vi "ATE_BSE_MAIN.vi"(8 "Error In":errorcluster) -> (0 "Error Out":errorcluster)   [LabVIEW 2021]
uses:
  Exit Event Handler/Controls/Exit Event Handle Comamnd.ctl
  Controls/ATE_BSE_Event_type_def.ctl
  Controls/ATE_BSE_Controls_ref.ctl
  Controls/ATE_BSE_ref_type_Def.ctl
  SubVI's/IP Simulation/Controls/IP_Cellular Tech Type def.ctl
  SubVI's/IP Simulation/Controls/IP_Network_Type def.ctl
  SubVI's/IP Simulation/Controls/IP_Type-Tydedef.ctl
  Controls/ATE_BSE_Queue_Operations.ctl
  APIs/Controls/TCP_FGV.ctl
  APIs/Controls/Base_Station_Emulator.ctl
  RE HIL/RE_Main/RE TCU HIL/Modules/Manual Mode/ATE_GE_Manual Mode_VI Ref Global Variable.vi
panel:
  in  "Configurations":enum32{"Configurations", "Main"}(tab)=enum."Main"
  in  "Configure":bool
  in  "Band":enum32{"GSM", "eNodeB", "gNodeB"}(tab)
  in  "GSM-Data":enum32{"SDR", "CELL", "PHY", "GPRS"}(tab)
  in  "GSM-SDR":T1={"DL Reference Power"=-13, "Serial Name"="", "UL Reference Power"=-13, "Radio Device"="0"} {"UL Reference Power" min=-64 max=-13; "DL Reference Power" min=-64 max=-13}
  in  "GSM-CELL":T2={"SMS Enabled"="0", "Eutra Operating Bands"="850", "Power Offset Indicator"="0", "Early Classmark Sending Control"="0", "Location Area Code"=1, "CALL Enabled"="0", "Loop Back Enabled"="1", "GPRS Enabled"="0", "SI Type 2 ter Indicator"="1", "ARFCN"=0, "Frequency Format ID"=71, "Mobile Country Code"=1, "Mobile Network Code"=1, "Cell Barred Access"="0", "Downlink Frequency"=0, "Uplink Frequency"=900200000} {"Mobile Network Code" min=0 max=999; "Mobile Country Code" min=0 max=99; "Frequency Format ID" min=0 max=1024; "ARFCN" min=0 max=1023; "Location Area Code" min=0 max=65535}
  in  "GSM-PHY":T3={"RACH Maximum Retransmission"="1", "RACH Transmission Slots"="14", "RACH Call Reestablishment"="1", "RACH Access Control Class"="0", "Block for Access Grant"="2", "Multiframe for Paging"="0", "Power Control Indicator"="0", "Radio Link Timeout"="15", "Cell Reselect Hysterisis"="3", "Attach/Detach Allowed"="1", "CCCH Combinations"="1", "t3212"=0, "DTX Indicator"="1", "Power Control Level"=0, "Minimum Received Signal Level"=0, "Half Rate Support"="0", "Add Reselect"="0"} {"Minimum Received Signal Level" min=0 max=63; "Power Control Level" min=0 max=31; "t3212" min=0 max=255}
  in  "GSM-GPRS":T4={"Priority Access THR"="6", "Acess Burst Type"="0", "Nack Countdown"="8", "BCCH/PDCH Measurement"="0", "Routing Area Code(RAC)"=128, "Network Control Order"="0", "t3168"="3", "t3192"="2", "Alpha"="10"}
  in  "eNodeB-Data":enum32{"SDR", "CELL", "PHY", "RRC"}(tab)
  in  "LTE-SDR":T5={"Radio Device"="0", "DL Reference Power"=-13, "Serail Name"="", "UL Reference Power"=-13, "DL Antennas"="1", "UL Antennas"="1"} {"UL Reference Power" min=-64 max=-13; "DL Reference Power" min=-64 max=-13}
  in  "LTE-CELL":T6={"Duplex Mode"="0", "Measurement Report"="1", "Eutra Operating Bands"="3", "Carrier Bandwidth"="10", "Physical Cell ID"=0, "Network Name"="MaxEye", "DL Frequency"=1842, "UL Frequency"=1747, "Transmission Mode"="TM1", "MNC Length"="2", "IMS Enabled"="0", "Tracking Area Code"=1, "Mobile Network Code"=1, "Mobile Country Code"=1} {"Mobile Country Code" min=0 max=99; "Mobile Network Code" min=0 max=999; "Tracking Area Code" min=0 max=65535; "Physical Cell ID" min=0 max=503}
  in  "LTE-PHY":T7={"PBCH Repetition"="0", "PUCCH Delta Shift"="1", "PUCCH CQI Number of RB"="0", "PHICH Resource"="ONESIXTH", "SRS Enable"="0", "PCCH Paging Cycle"="256", "BCCH Modification Coefficient"="2", "PUSCH Alpha"="1", "PUSCH DMRS Enable"="0", "PHICH Duration"="0", "PUCCH HARQ Max Transmission"=4, "PCCH Narrowband Count"="2", "PUSCH Power Offset"=-96, "PUCCH Power Offset"=-96, "PDSCH Power Boost"="0", "PUCCH An Occassions"="0", "PUUCH CS Antenna Ports"="1", "PRACH Response Window Size"="10", "PRACH Contention Resolution Timer"="48", "PRACH Ramping Step Size"="4", "PDSCH Reference Power"=-27, "PRACH Root Sequence Index"=0, "PRACH Maximum Transmissions"="10", "PRACH Initial Received Target Power"="-108", "PRACH Configuration Index"=0} {"PRACH Configuration Index" min=0 max=63; "PRACH Root Sequence Index" min=0 max=837; "PDSCH Reference Power" min=-70 max=0; "PUCCH Power Offset" min=-127 max=-96; "PUSCH Power Offset" min=-126 max=24; "PUCCH HARQ Max Transmission" min=0 max=16}
  in  "LTE-RRC":T8={"RLC Maximum Retransmision Threshold"="4", "RLC Timer Poll Retransmit"=80, "RLC Timer Reordering"=35, "RLC Timer Status Prohibit"=0, "RLC Poll PDU"=4, "RLC Poll Byte"=25} {"RLC Poll Byte" min=0 step=25; "RLC Poll PDU" min=0 step=4; "RLC Timer Status Prohibit" min=0 max=500 step=5; "RLC Timer Reordering" min=0 max=200 step=5; "RLC Timer Poll Retransmit" min=0 max=500 step=5}
  in  "gNodeB-Data":enum32{"SDR", "CELL", "PHY", "RRC"}(tab)
  in  "NR-SDR":T9={"DL Reference Power"=-13, "Serail Name"="", "UL Reference Power"=-13, "DL Antennas"="1", "UL Antennas"="1", "Radio Device"="0"} {"UL Reference Power" min=-64 max=-13; "DL Reference Power" min=-64 max=-13}
  in  "NR-CELL":T10={"Tracking Area Code"=1, "Mobile Country Code"=1, "Mobile Network Code"=1, "Operating Bands"="77", "Physical Cell ID"=0, "DL Offset to Carrier"=0, "Subcarrier Spacing"="1", "UL Offset to Carrier 2"=0, "Carrier Bandwidth"="10", "Transmission Mode"="TM1", "CSI-RS"="1", "SRS"="1", "Measurement Report"="1"} {"Physical Cell ID" min=0 max=503; "Mobile Network Code" min=0 max=999; "Mobile Country Code" min=0 max=99; "Tracking Area Code" min=0 max=65535}
  in  "NR-PHY":T11={"PDSCH Reference Power"=-27, "SSB RSRP Threshold"=-109, "PRACH Contention Resolution Timer"=7, "Preamble Per SSB"=14, "Preamble Per SSB Format"=4, "UE Power Level Grant"=-90, "RA Response Window"="10", "Power Ramp Step Size"="2", "Preamble Root Sequence Index"="139", "Preamble Transmission Count"="10", "Preamble Received Power"=-96, "Zero Correlation Zone Configuration"=13, "Msg Frequency Division Multiplexing"="one", "PRACH Configuration Index"=98, "Preamble Timing Offset"=1, "Preamble Format"=0, "Resource Restriction Type"="0"} {"Preamble Format" min=0 max=3; "Preamble Timing Offset" min=-1 max=6; "PRACH Configuration Index" min=0 max=255; "Zero Correlation Zone Configuration" min=1 max=15; "Preamble Received Power" min=-202 max=-60; "UE Power Level Grant" min=-202 max=24; "Preamble Per SSB Format" min=0 max=7; "Preamble Per SSB" min=1 max=16; "PRACH Contention Resolution Timer" min=0 max=7; "SSB RSRP Threshold" min=-140 max=-90; "PDSCH Reference Power" min=-70 max=0}
  in  "NR-RRC":T12={"Ciphering Algorithms for SRB"="0", "Integrity Algorithms for SRB"="0", "Ciphering Algorithms for DRB"="1", "Integrity Algorithms for DRB"="1"}
  in  "Cancel Configurations":bool
  in  "Sim Configurations":bool
  in  "SelectNetwork2":cluster{"Nw1-check":bool, "NW-Combo":string}={"Nw1-check"=FALSE, "NW-Combo"="GSM"}
  in  "SelectNetwork1":cluster{"Nw1-check":bool, "NW-Combo":string}={"Nw1-check"=FALSE, "NW-Combo"="GSM"}
  in  "SelectNetwork3":cluster{"Nw1-check":bool, "NW-Combo":string}={"Nw1-check"=FALSE, "NW-Combo"="GSM"}
  in  "WWW":bool
  in  "IMS":bool
  in  "ECall":bool
  in  "UE4":bool
  in  "UE3":bool
  in  "UE2":bool
  in  "UE1":bool
  out "Trace_Table2":i32(listbox)
  out "Trace_Table1":i32(listbox)
  out "Status":string
  in  "IP simulation":bool
  in  "Start":bool
  in  "Reset":bool
  in  "Download":bool
  in  "Upload":bool
  out "UE - 4":T13
  out "UE - 3":T14
  out "UE - 2":T15
  out "UE - 1":T16
  out "Network-1":T17
  out "Network-2":T18
  out "Network-3":T19
  out "Time Stamp":timestamp format="%<%H:%M:%S>T"
  # "Cellular Network Emulator"
  # "BASE STATION :"
  # "CONFIGURATIONS"
  # "Power Level"
  # "Frequency"
  # "Throughput"
  # "Downlink"
  # "Uplink"
  # "NETWORK - 1"
  # "Power Level"
  # "Frequency"
  # "Throughput"
  # "Downlink"
  # "Uplink"
  # "NETWORK - 2"
  # "Power Level"
  # "Frequency"
  # "Throughput"
  # "Downlink"
  # "Uplink"
  # "NETWORK - 3"
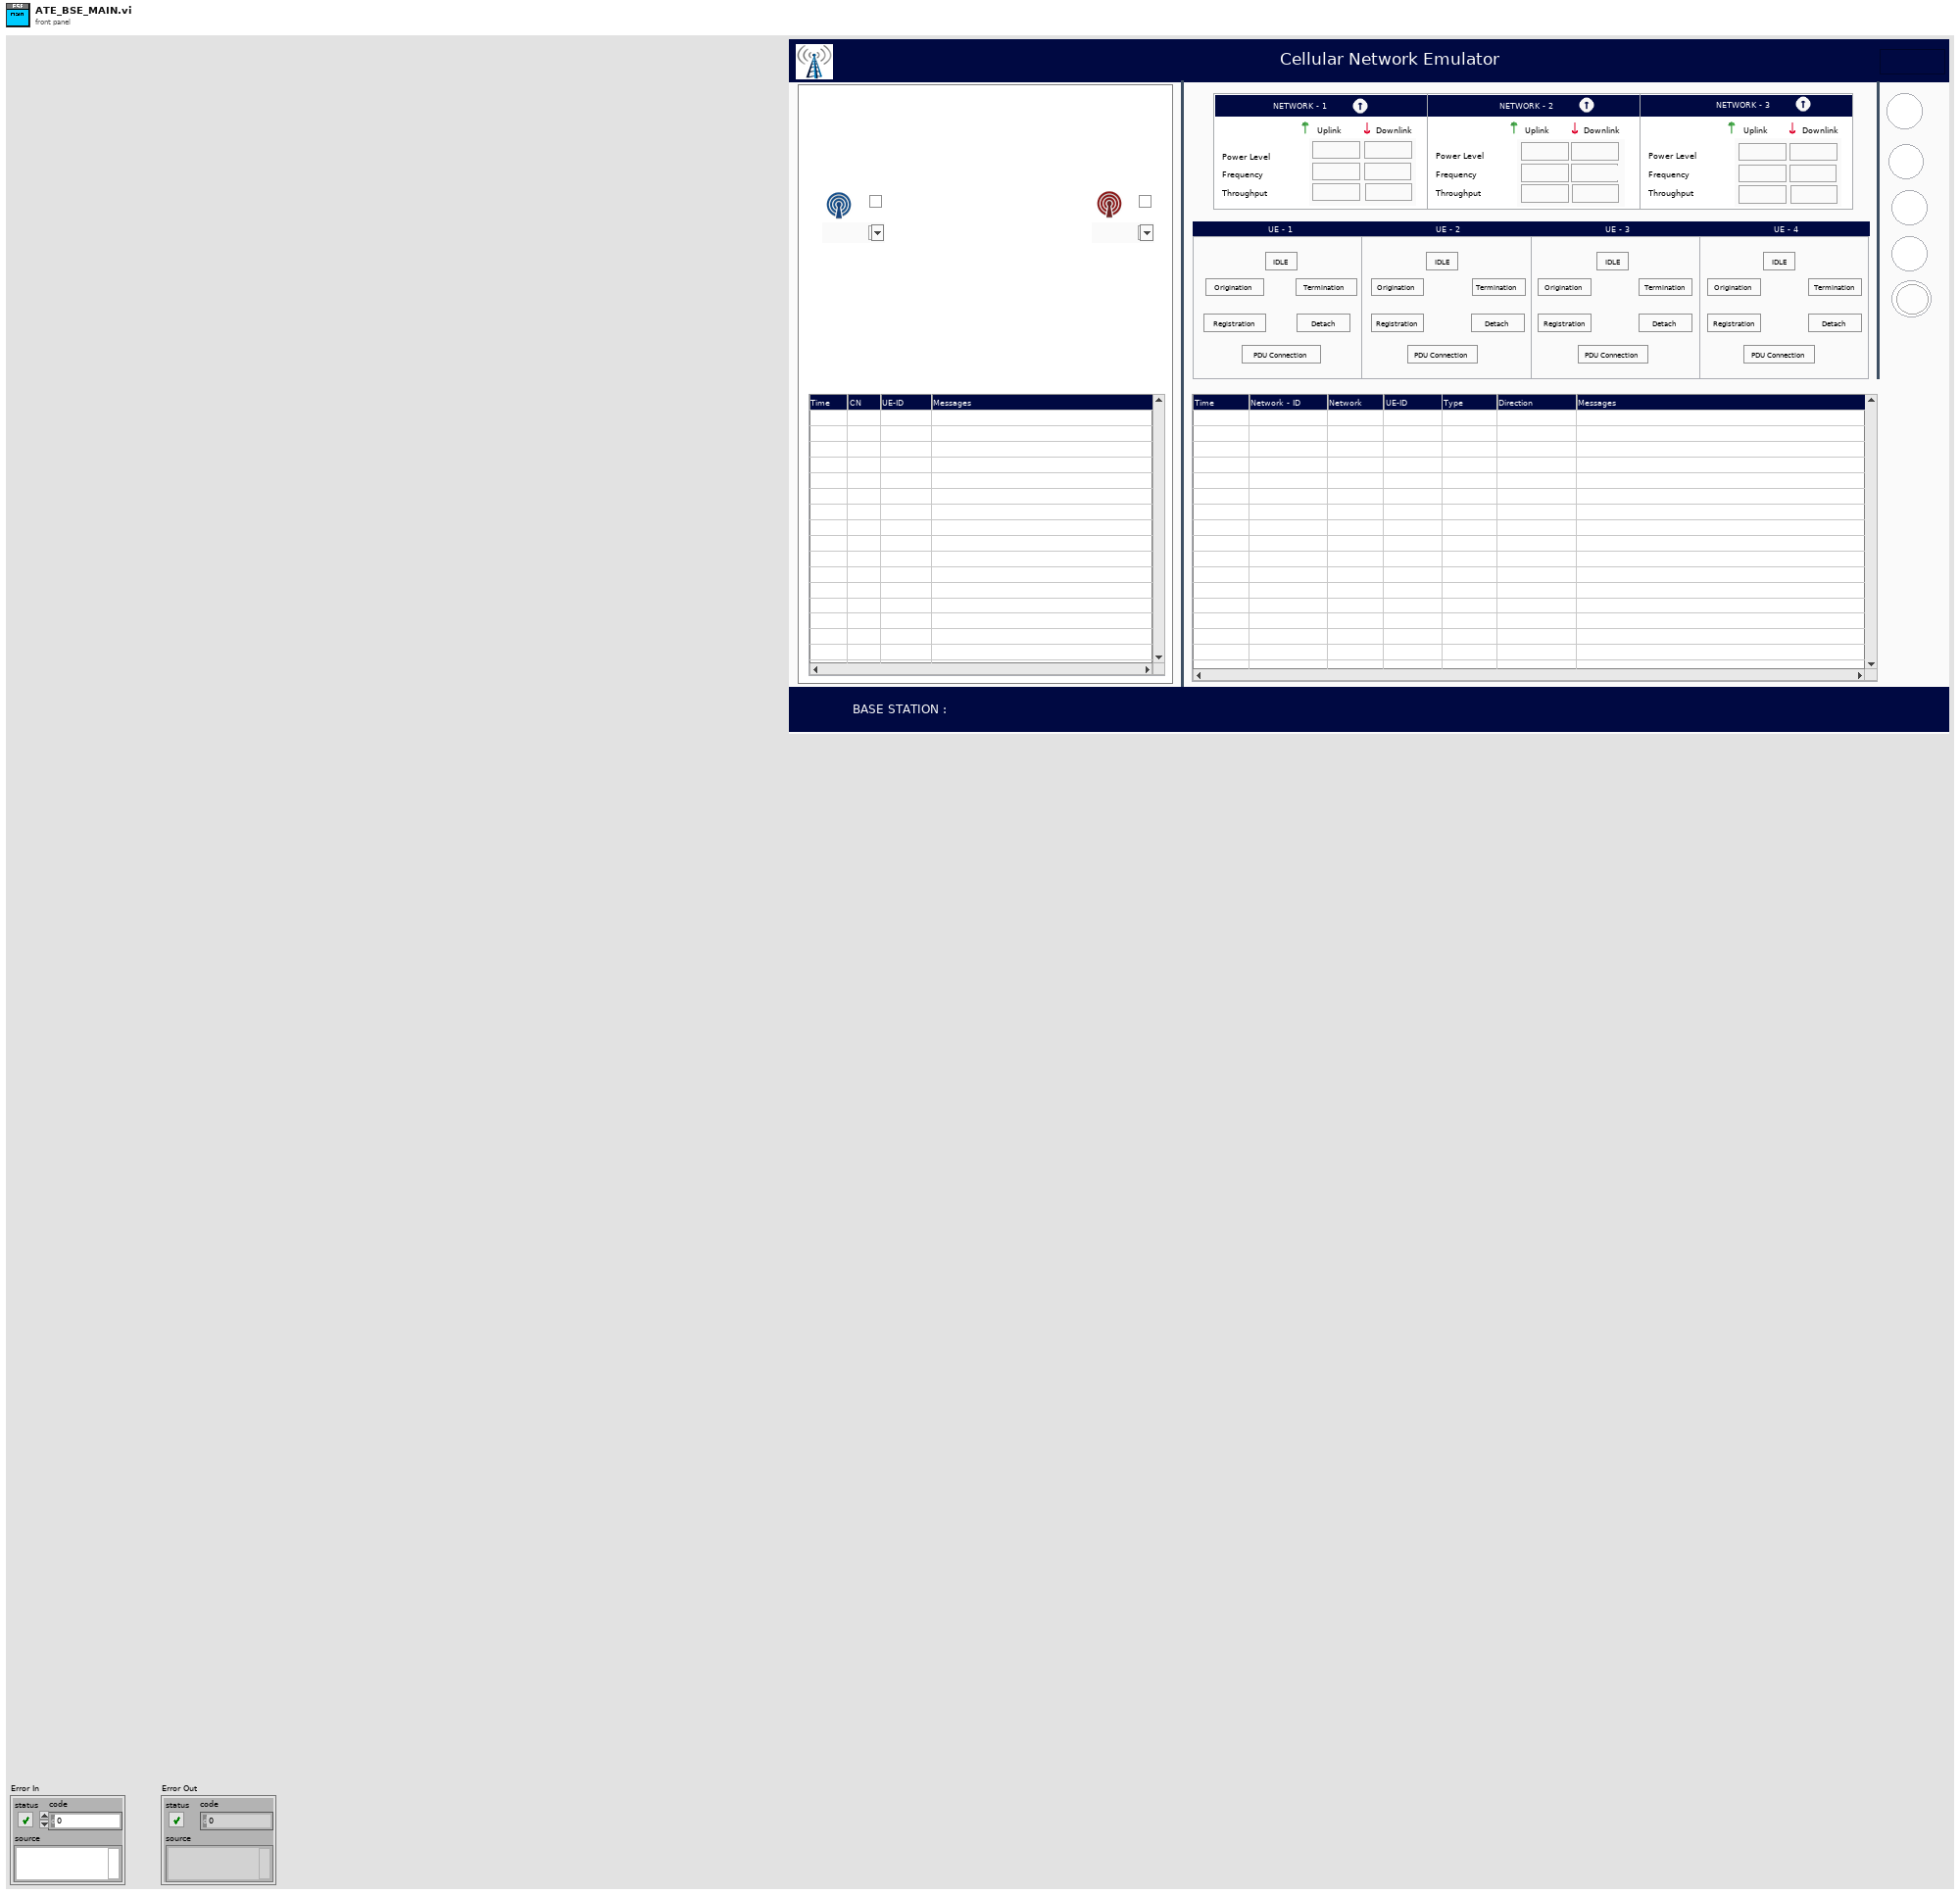
[diagram p1: front panel]
types:
  T1 = cluster{"DL Reference Power":i32, "Serial Name":string, "UL Reference Power":i32, "Radio Device":string}
  T2 = cluster{"SMS Enabled":string, "Eutra Operating Bands":string, "Power Offset Indicator":string, "Early Classmark Sending Control":string, "Location Area Code":i32, "CALL Enabled":string, "Loop Back Enabled":string, "GPRS Enabled":string, "SI Type 2 ter Indicator":string, "ARFCN":i64, "Frequency Format ID":i64, "Mobile Country Code":i64, "Mobile Network Code":i64, "Cell Barred Access":string, "Downlink Frequency":i32, "Uplink Frequency":i32}
  T3 = cluster{"RACH Maximum Retransmission":string, "RACH Transmission Slots":string, "RACH Call Reestablishment":string, "RACH Access Control Class":string, "Block for Access Grant":string, "Multiframe for Paging":string, "Power Control Indicator":string, "Radio Link Timeout":string, "Cell Reselect Hysterisis":string, "Attach/Detach Allowed":string, "CCCH Combinations":string, "t3212":i64, "DTX Indicator":string, "Power Control Level":i64, "Minimum Received Signal Level":i64, "Half Rate Support":string, "Add Reselect":string}
  T4 = cluster{"Priority Access THR":string, "Acess Burst Type":string, "Nack Countdown":string, "BCCH/PDCH Measurement":string, "Routing Area Code(RAC)":i32, "Network Control Order":string, "t3168":string, "t3192":string, "Alpha":string}
  T5 = cluster{"Radio Device":string, "DL Reference Power":i32, "Serail Name":string, "UL Reference Power":i32, "DL Antennas":string, "UL Antennas":string}
  T6 = cluster{"Duplex Mode":string, "Measurement Report":string, "Eutra Operating Bands":string, "Carrier Bandwidth":string, "Physical Cell ID":i64, "Network Name":string, "DL Frequency":i32, "UL Frequency":i32, "Transmission Mode":string, "MNC Length":string, "IMS Enabled":string, "Tracking Area Code":i32, "Mobile Network Code":i32, "Mobile Country Code":i32}
  T7 = cluster{"PBCH Repetition":string, "PUCCH Delta Shift":string, "PUCCH CQI Number of RB":string, "PHICH Resource":string, "SRS Enable":string, "PCCH Paging Cycle":string, "BCCH Modification Coefficient":string, "PUSCH Alpha":string, "PUSCH DMRS Enable":string, "PHICH Duration":string, "PUCCH HARQ Max Transmission":i64, "PCCH Narrowband Count":string, "PUSCH Power Offset":i64, "PUCCH Power Offset":i64, "PDSCH Power Boost":string, "PUCCH An Occassions":string, "PUUCH CS Antenna Ports":string, "PRACH Response Window Size":string, "PRACH Contention Resolution Timer":string, "PRACH Ramping Step Size":string, "PDSCH Reference Power":i64, "PRACH Root Sequence Index":i64, "PRACH Maximum Transmissions":string, "PRACH Initial Received Target Power":string, "PRACH Configuration Index":i64}
  T8 = cluster{"RLC Maximum Retransmision Threshold":string, "RLC Timer Poll Retransmit":i32, "RLC Timer Reordering":i32, "RLC Timer Status Prohibit":i32, "RLC Poll PDU":i32, "RLC Poll Byte":i32}
  T9 = cluster{"DL Reference Power":i32, "Serail Name":string, "UL Reference Power":i32, "DL Antennas":string, "UL Antennas":string, "Radio Device":string}
  T10 = cluster{"Tracking Area Code":i64, "Mobile Country Code":i64, "Mobile Network Code":i64, "Operating Bands":string, "Physical Cell ID":i64, "DL Offset to Carrier":i32, "Subcarrier Spacing":string, "UL Offset to Carrier 2":i32, "Carrier Bandwidth":string, "Transmission Mode":string, "CSI-RS":string, "SRS":string, "Measurement Report":string}
  T11 = cluster{"PDSCH Reference Power":i64, "SSB RSRP Threshold":i64, "PRACH Contention Resolution Timer":i64, "Preamble Per SSB":i64, "Preamble Per SSB Format":i64, "UE Power Level Grant":i64, "RA Response Window":string, "Power Ramp Step Size":string, "Preamble Root Sequence Index":string, "Preamble Transmission Count":string, "Preamble Received Power":i64, "Zero Correlation Zone Configuration":i64, "Msg Frequency Division Multiplexing":string, "PRACH Configuration Index":i64, "Preamble Timing Offset":i64, "Preamble Format":i64, "Resource Restriction Type":string}
  T12 = cluster{"Ciphering Algorithms for SRB":string, "Integrity Algorithms for SRB":string, "Ciphering Algorithms for DRB":string, "Integrity Algorithms for DRB":string}
  T13 = cluster{"UE4-Idle":bool, "UE4-Origination":bool, "UE4-Registration":bool, "UE4-Pdu Connection":bool, "UE4-Termination":bool, "UE4-Detach":bool}
  T14 = cluster{"UE3-Idle":bool, "UE3-Origination":bool, "UE3-Registration":bool, "UE3-Pdu Connection":bool, "UE3-Termination":bool, "UE3-Detach":bool}
  T15 = cluster{"UE2-Idle":bool, "UE2-Origination":bool, "UE2-Registration":bool, "UE2-Pdu Connection":bool, "UE2-Termination":bool, "UE2-Detach":bool}
  T16 = cluster{"UE1-Idle":bool, "UE1-Origination":bool, "UE1-Registration":bool, "UE1-Pdu Connection":bool, "UE1-Termination":bool, "UE1-Detach":bool}
  T17 = cluster{"NW1-Thr-Down":dbl, "NW1-Thr-Up":dbl, "NW1-Fre-Down":dbl, "NW1-Fre-Up":dbl, "NW1-PwL-Down":dbl, "NW1-PwL-Up":dbl}
  T18 = cluster{"NW2-Thr-Down":dbl, "NW2-Thr-Up":dbl, "NW2-Fre-Down":dbl, "NW2-Fre-Up":dbl, "NW2-PwL-Down":dbl, "NW2-PwL-Up":dbl}
  T19 = cluster{"NW3-Thr-Down":dbl, "NW3-Thr-Up":dbl, "NW3-Fre-Down":dbl, "NW3-Fre-Up":dbl, "NW3-PwL-Down":dbl, "NW3-PwL-Up":dbl}
  T20 = typedef "ATE_BSE_Queue_Operations.ctl" = enum16{"Init", "Get Queue", "Flush", "Close"}
  T21 = typedef "ATE_BSE_Controls_ref.ctl" = cluster{"Ref_Cluster":T22, "Time Stamp":timestamp, "Network-3":cluster{"NW3-Thr-Down":dbl, "NW3-Thr-Up":dbl, "NW3-Fre-Down":dbl, "NW3-Fre-Up":dbl, "NW3-PwL-Down":dbl, "NW3-PwL-Up":dbl}, "Network-2":cluster{"NW2-Thr-Down":dbl, "NW2-Thr-Up":dbl, "NW2-Fre-Down":dbl, "NW2-Fre-Up":dbl, "NW2-PwL-Down":dbl, "NW2-PwL-Up":dbl}, "Network-1":cluster{"NW1-Thr-Down":dbl, "NW1-Thr-Up":dbl, "NW1-Fre-Down":dbl, "NW1-Fre-Up":dbl, "NW1-PwL-Down":dbl, "NW1-PwL-Up":dbl}, "UE - 4":cluster{"UE4-Idle":bool, "UE4-Origination":bool, "UE4-Registration":bool, "UE4-Pdu Connection":bool, "UE4-Termination":bool, "UE4-Detach":bool}, "UE - 2":cluster{"UE2-Idle":bool, "UE2-Origination":bool, "UE2-Registration":bool, "UE2-Pdu Connection":bool, "UE2-Termination":bool, "UE2-Detach":bool}, "UE - 1":cluster{"UE1-Idle":bool, "UE1-Origination":bool, "UE1-Registration":bool, "UE1-Pdu Connection":bool, "UE1-Termination":bool, "UE1-Detach":bool}, "UE - 3":cluster{"UE3-Idle":bool, "UE3-Origination":bool, "UE3-Registration":bool, "UE3-Pdu Connection":bool, "UE3-Termination":bool, "UE3-Detach":bool}, "IP simulation":bool, "Stop":bool, "Reset":bool, "Download":bool, "Upload":bool, "UE4":bool, "UE3":bool, "UE2":bool, "UE1":bool, "Trace_Table1":i32, "Status":string, "Trace_Table2":i32, "SelectNetwork1":cluster{"Nw1-check":bool, "NW-Combo":string}, "SelectNetwork2":cluster{"Nw1-check":bool, "NW-Combo":string}, "SelectNetwork3":cluster{"Nw1-check":bool, "NW-Combo":string}, "IMS":bool, "WWW":bool, "Sim Configuration":bool, "Ecall":bool, "Configurations":enum32{"Configurations", "Main"}, "Band":enum32{"GSM", "gNodeB", "eNodeB"}, "GSM-Data":enum32{"SDR", "CELL", "PHY", "GPRS"}, "eNodeB-Data":enum32{"SDR", "CELL", "PHY", "RRC"}, "gNodeB-Data":enum32{"SDR", "CELL", "PHY", "RRC"}, "Cancel Configurations":bool, "GSM-SDR":cluster{"DL Reference Power":i32, "Serail Name":string, "UL Reference Power":i32, "Radio Device":string}, "GSM-PHY":cluster{"RACH Maximum Retransmission":string, "RACH Transmission Slots":string, "RACH Call Reestablishment":string, "RACH Access Control Class":string, "Block for Access Grant":string, "Multiframe for Paging":string, "Power Control Indicator":string, "Radio Link Timeout":string, "Cell Reselect Hysterisis":string, "Attach/Detach Allowed":string, "CCCH Combinations":string, "t3212":i64, "DTX Indicator":string, "Power Control Level":i64, "Minimum Received Signal Level":i64, "Half Rate Support":string, "Add Reselect":string}, "GSM-CELL":cluster{"SMS Enabled":string, "Eutra Operating Bands":string, "Power Offset Indicator":string, "Early Classmark Sending Control":string, "Location Area Code":i32, "CALL Enabled":string, "Loop Back Enabled":string, "GPRS Enabled":string, "SI Type 2 ter Indicator":string, "ARFCN":i64, "Frequency Format ID":i64, "Mobile Country Code":i64, "Mobile Network Code":i64, "Cell Barred Access":string, "Downlink Frequency":i32, "Uplink Frequency":i32}, "GSM-GPRS":cluster{"Priority Access THR":string, "Acess Burst Type":string, "Nack Countdown":string, "BCCH/PDCH Measurement":string, "Routing Area Code(RAC)":i32, "Network Control Order":string, "t3168":string, "t3192":string, "Alpha":string}, "LTE-SDR":cluster{"Radio Device":string, "DL Reference Power":i32, "Serail Name":string, "UL Reference Power":i32, "DL Antennas":string, "UL Antennas":string}, "LTE-PHY":cluster{"PBCH Repetition":string, "PUCCH Delta Shift":string, "PUCCH CQI Number of RB":string, "PHICH Resource":string, "SRS Enable":string, "PCCH Paging Cycle":string, "BCCH Modification Coefficient":string, "PUSCH Alpha":string, "PUSCH DMRS Enable":string, "PHICH Duration":string, "PUCCH HARQ Max Transmission":i64, "PCCH Narrowband Count":string, "PUSCH Power Offset":i64, "PUCCH Power Offset":i64, "PDSCH Power Boost":string, "PUCCH An Occassions":string, "PUUCH CS Antenna Ports":string, "PRACH Response Window Size":string, "PRACH Contention Resolution Timer":string, "PRACH Ramping Step Size":string, "PDSCH Reference Power":i64, "PRACH Root Sequence Index":i64, "PRACH Maximum Transmissions":string, "PRACH Initial Received Target Power":string, "PRACH Configuration Index":i64}, "LTE-CELL":cluster{"Duplex Mode":string, "Measurement Report":string, "Eutra Operating Bands":string, "Carrier Bandwidth":string, "Physical Cell ID":i64, "Network Name":string, "DL Frequency":i32, "UL Frequency":i32, "Transmission Mode":string, "MNC Length":string, "IMS Enabled":string, "Tracking Area Code":i32, "Mobile Network Code":i32, "Mobile Country Code":i32}, "LTE-RRC":cluster{"RLC Maximum Retransmision Threshold":string, "RLC Timer Poll Retransmit":i32, "RLC Timer Reordering":i32, "RLC Timer Status Prohibit":i32, "RLC Poll PDU":i32, "RLC Poll Byte":i32}, "NR-SDR":cluster{"DL Reference Power":i32, "Serail Name":string, "UL Reference Power":i32, "DL Antennas":string, "UL Antennas":string, "Radio Device":string}, "NR-PHY":cluster{"PDSCH Reference Power":i64, "SSB RSRP Threshold":i64, "PRACH Contention Resolution Timer":i64, "Preamble Per SSB":i64, "Preamble Per SSB Format":i64, "UE Power Level Grant":i64, "RA Response Window":string, "Power Ramp Step Size":string, "Preamble Root Sequence Index":string, "Preamble Transmission Count":string, "Preamble Received Power":i64, "Zero Correlation Zone Configuration":i64, "Msg Frequency Division Multiplexing":string, "PRACH Configuration Index":i64, "Preamble Timing Offset":i64, "Preamble Format":i64, "Resource Restriction Type":string}, "NR-CELL":cluster{"Tracking Area Code":i64, "Mobile Country Code":i64, "Mobile Network Code":i64, "Operating Bands":string, "Physical Cell ID":i64, "DL Offset to Carrier":i32, "Subcarrier Spacing":string, "UL Offset to Carrier 2":i32, "Carrier Bandwidth":string, "Transmission Mode":string, "CSI-RS":string, "SRS":string, "Measurement Report":string}, "NR-RRC":cluster{"Ciphering Algorithms for SRB":string, "Integrity Algorithms for SRB":string, "Ciphering Algorithms for DRB":string, "Integrity Algorithms for DRB":string}, "IP_UI":cluster{"Add":bool, "Close":bool, "IP_UI":cluster{"Cellular Tect":T23, "IP_NETWORK":T24, "IP_TYPE":T25, "IP_Client Address":string, "IP_ThgroughPut(Mbps)":i32, "Duration":i32, "Run":bool}[]}, "IMS_DATA":string[][], "ECall DATA":string[][]}
  T22 = typedef "ATE_BSE_ref_type_Def.ctl" = cluster{"UE1":refnum<vi>, "UE2":refnum<vi>, "UE3":refnum<vi>, "SelectNetwork1":refnum<vi>, "SelectNetwork3":refnum<vi>, "SelectNetwork2":refnum<vi>, "Trace_Table1":refnum<vi>, "UE - 1":refnum<vi>, "UE - 2":refnum<vi>, "UE - 3":refnum<vi>, "UE - 4":refnum<vi>, "Network-3":refnum<vi>, "Status":refnum<vi>, "Trace_Table2":refnum<vi>, "UE4":refnum<vi>, "Stop":refnum<vi>, "Reset":refnum<vi>, "IP simulation":refnum<vi>, "Upload":refnum<vi>, "Download":refnum<vi>, "Network-1":refnum<vi>, "Time Stamp":refnum<vi>, "Network-2":refnum<vi>, "IMS":refnum<vi>, "GSM-Data":refnum<vi>, "Configurations":refnum<vi>, "Band":refnum<vi>, "Sim Configurations":refnum<vi>, "ECall":refnum<vi>, "WWW":refnum<vi>, "Cancel Configurations":refnum<vi>, "GSM-PHY":refnum<vi>, "GSM-CELL":refnum<vi>, "GSM-GPRS":refnum<vi>, "LTE-CELL":refnum<vi>, "LTE-PHY":refnum<vi>, "LTE-RRC":refnum<vi>, "LTE-SDR":refnum<vi>, "NR-RRC":refnum<vi>, "NR-SDR":refnum<vi>, "NR-PHY":refnum<vi>, "NR-CELL":refnum<vi>, "GSM-SDR":refnum<vi>, "gNodeB-Data":refnum<vi>, "eNodeB-Data":refnum<vi>}
  T23 = typedef "IP_Cellular Tech Type def.ctl" = string
  T24 = typedef "IP_Network_Type def.ctl" = string
  T25 = typedef "IP_Type-Tydedef.ctl" = string
  T26 = typedef "ATE_BSE_Event_type_def.ctl" = enum16{"Initialize", "Configure", "Ip Simulation", "IMS", "ECall", "Start Base Station", "Exit", "Error"}
  T27 = typedef "Exit Event Handle Comamnd.ctl" = enum16{"Init", "Close", "Generate Event"}
  T28 = cluster{"Cellular Tect":T23, "IP_NETWORK":T24, "IP_TYPE":T25, "IP_Client Address":string, "IP_ThgroughPut(Mbps)":i32, "Duration":i32, "Run":bool}[]
  T29 = typedef "TCP_FGV.ctl" = enum16{"Open", "Read", "Write", "Close"}
  T30 = typedef "Base_Station_Emulator.ctl" = string
  T31 = cluster{"Add":bool, "Close":bool, "IP_UI":cluster{"Cellular Tect":T23, "IP_NETWORK":T24, "IP_TYPE":T25, "IP_Client Address":string, "IP_ThgroughPut(Mbps)":i32, "Duration":i32, "Run":bool}[]}
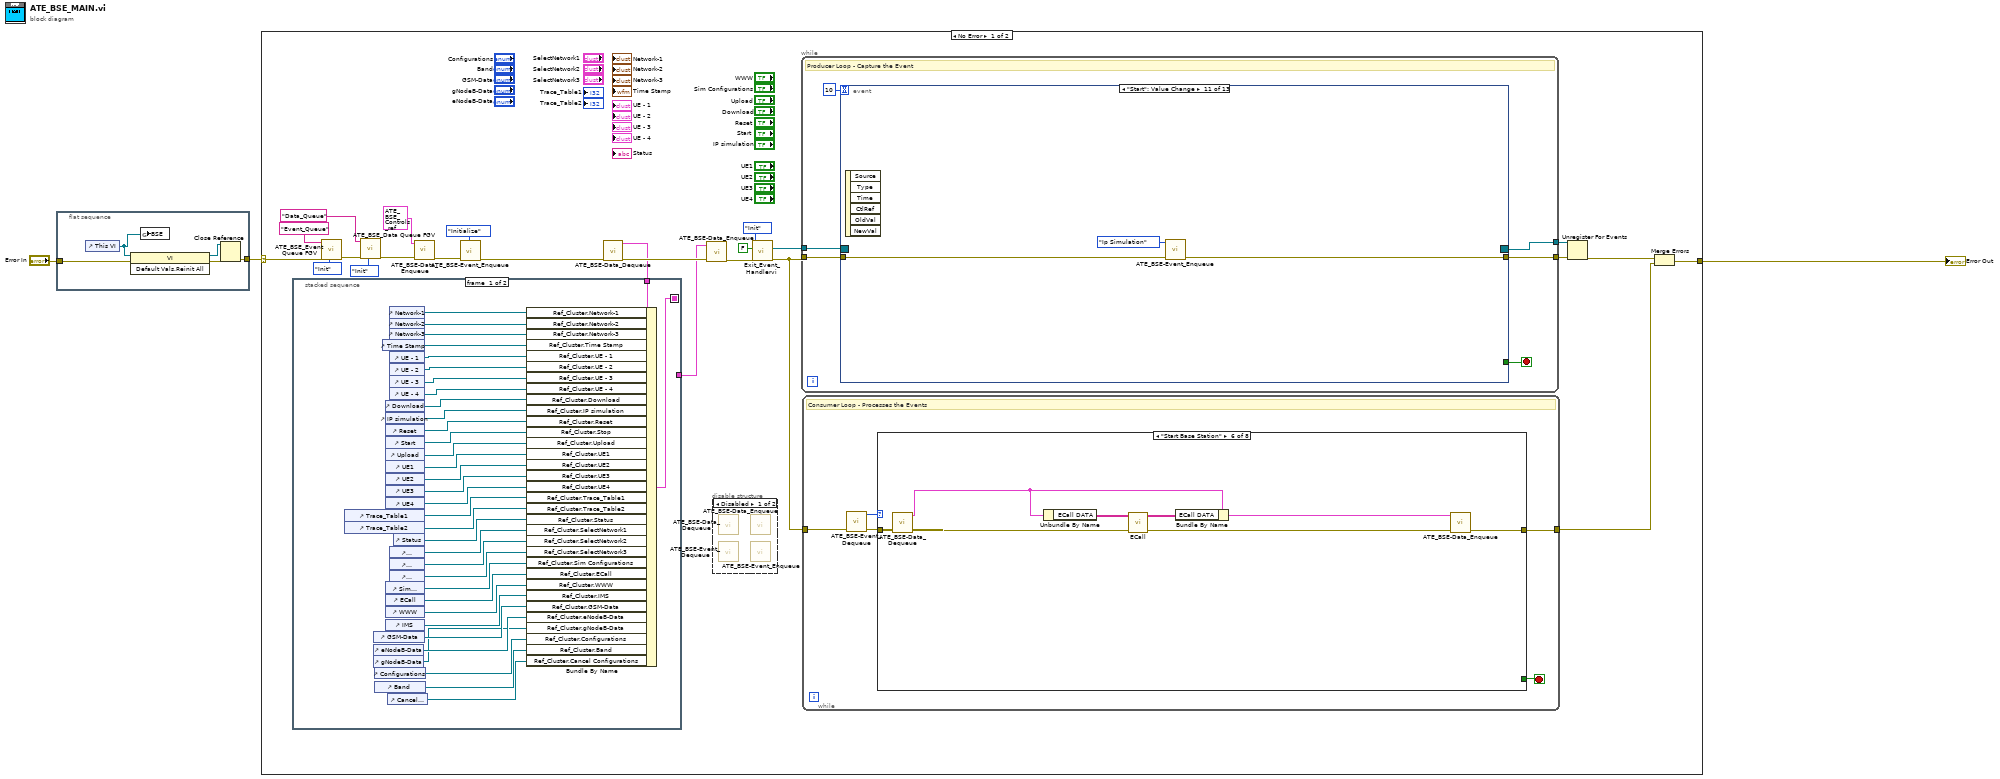
[diagram p0: block diagram]
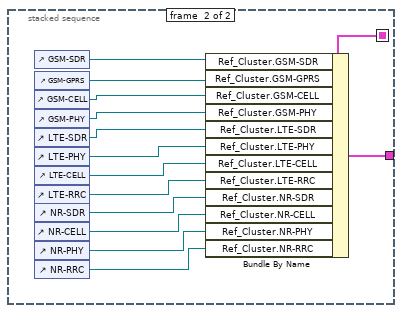
[diagram p2: hidden frame]
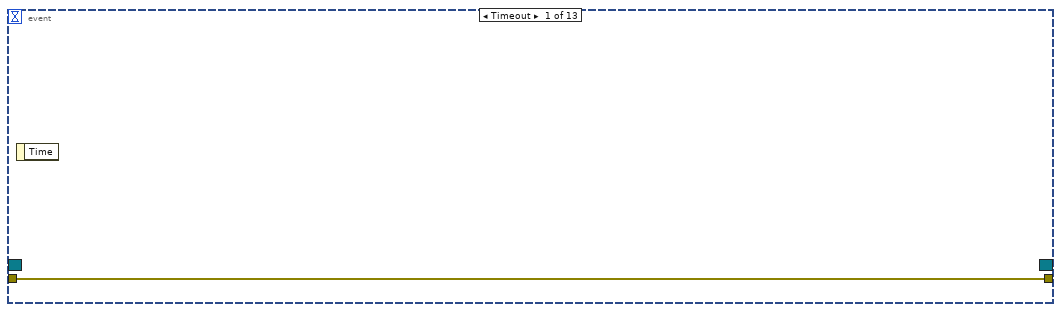
[diagram p4: hidden frame]
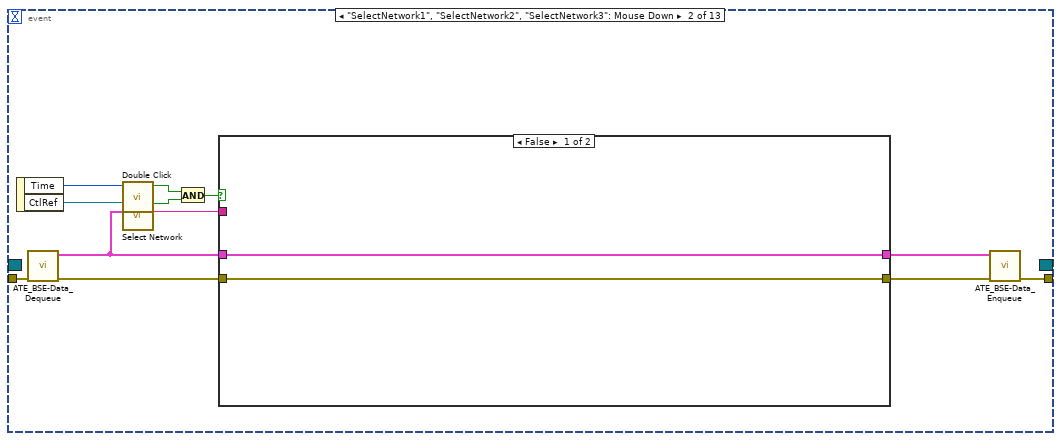
[diagram p5: hidden frame]
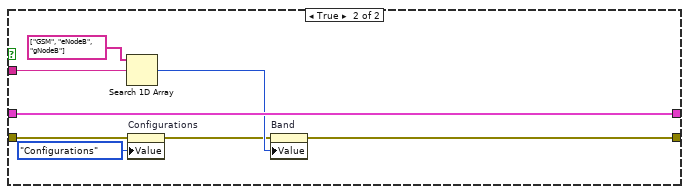
[diagram p6: hidden frame]
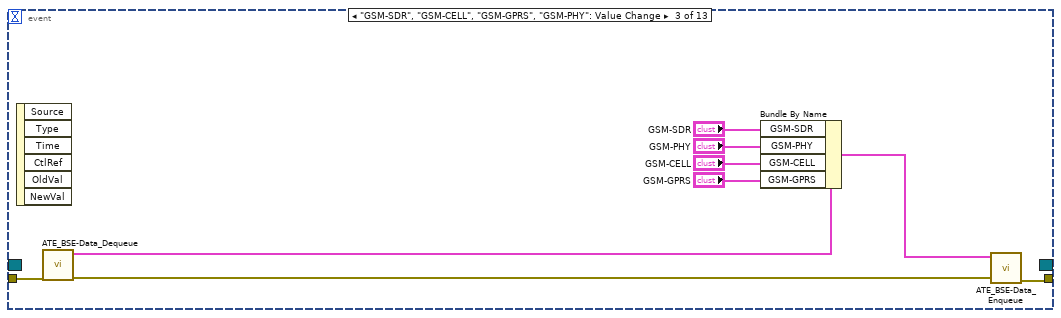
[diagram p7: hidden frame]
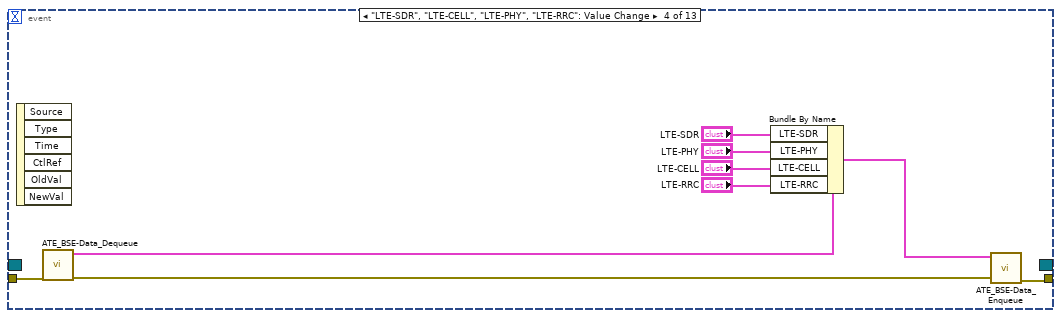
[diagram p8: hidden frame]
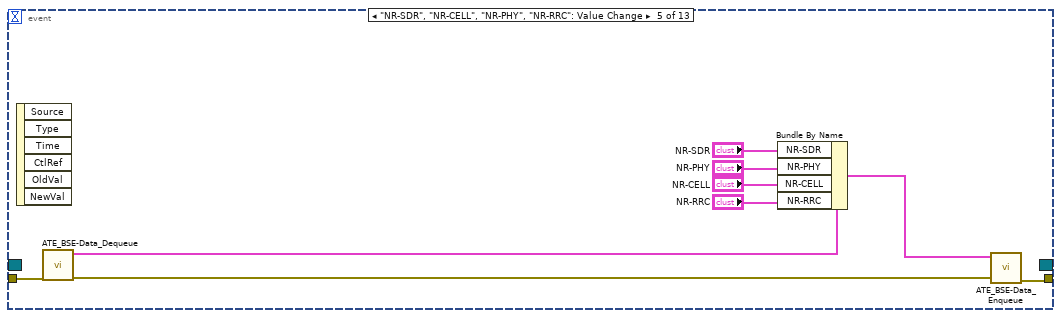
[diagram p9: hidden frame]
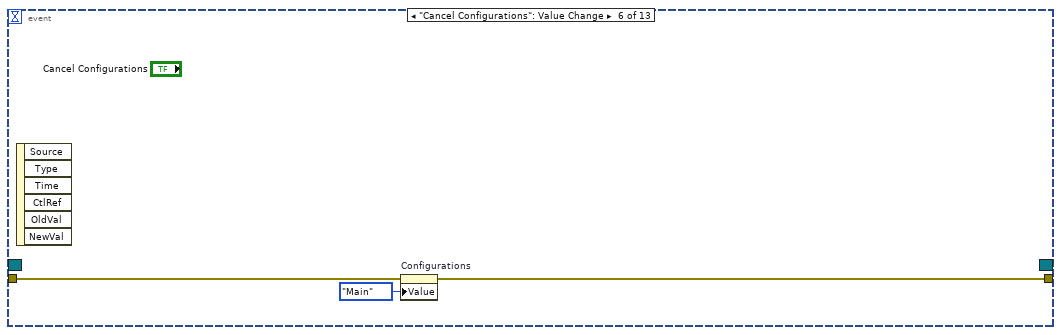
[diagram p10: hidden frame]
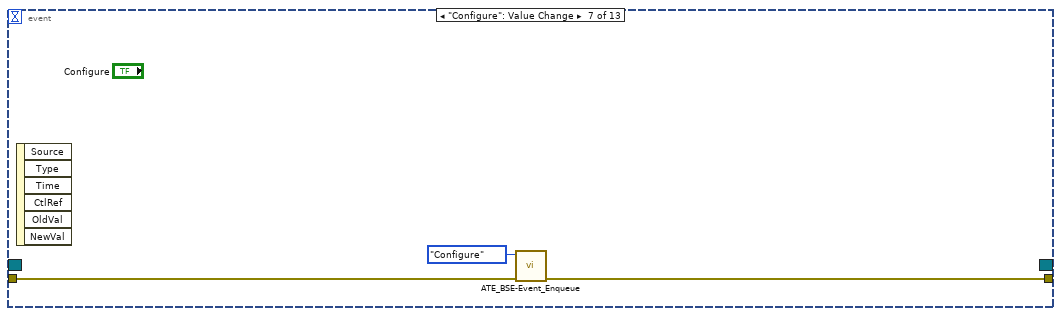
[diagram p11: hidden frame]
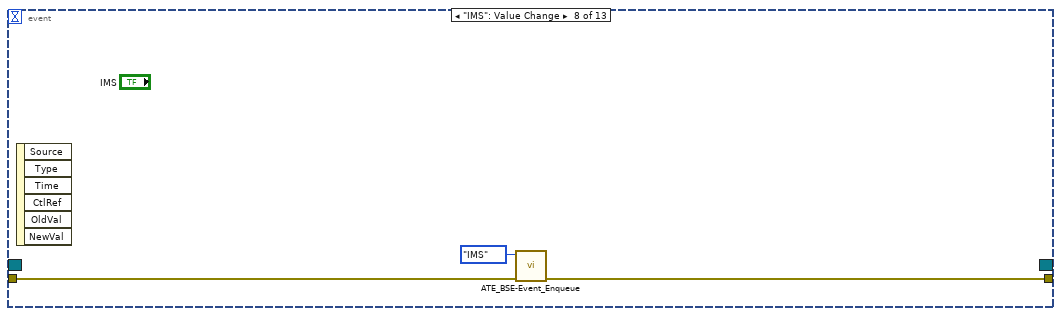
[diagram p12: hidden frame]
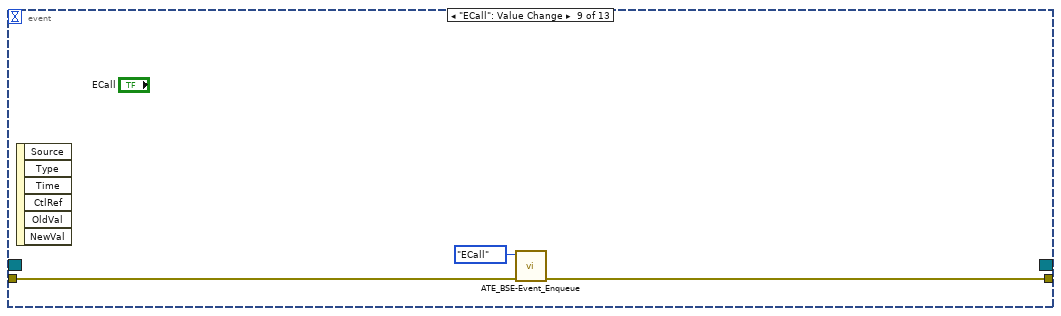
[diagram p13: hidden frame]
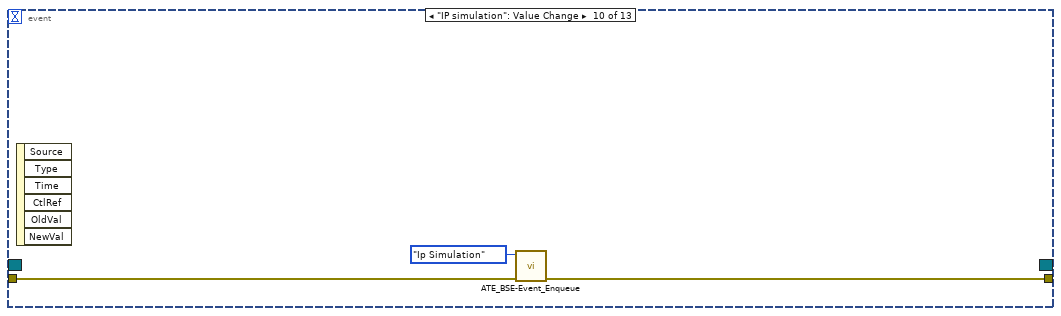
[diagram p14: hidden frame]
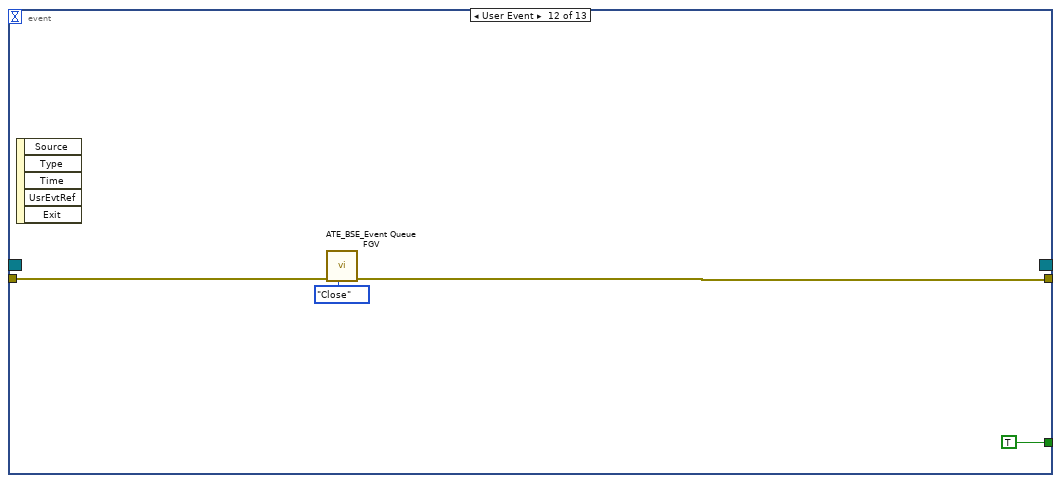
[diagram p15: hidden frame]
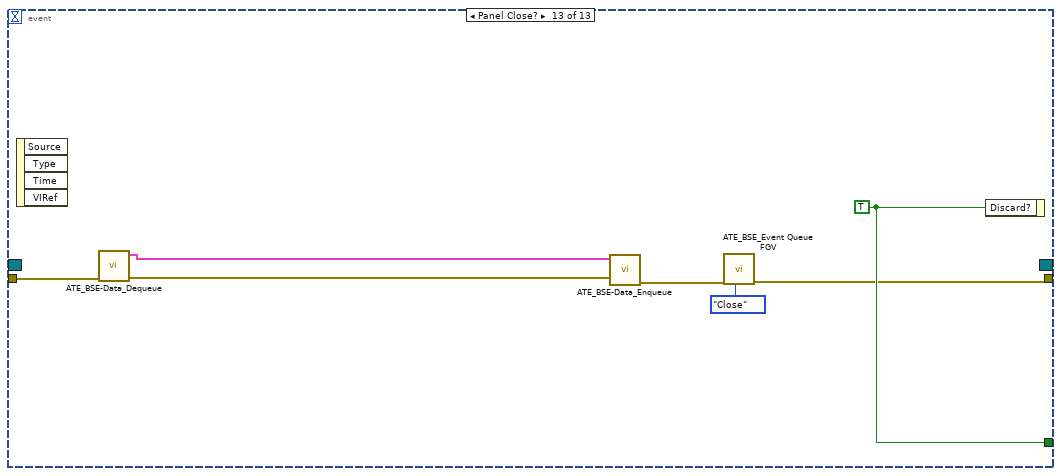
[diagram p16: hidden frame]
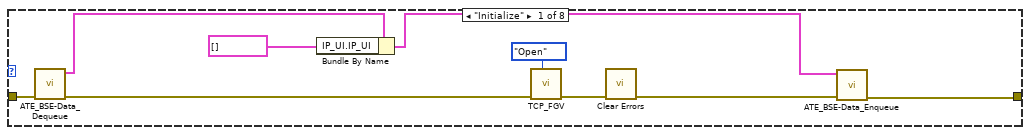
[diagram p17: hidden frame]
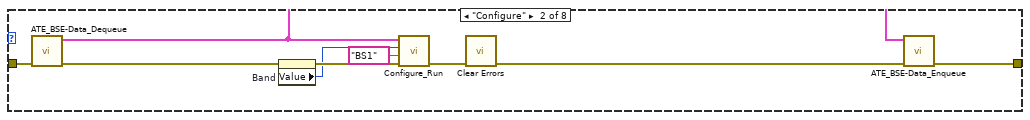
[diagram p18: hidden frame]
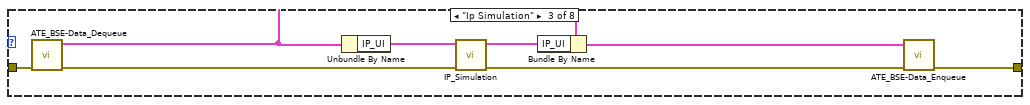
[diagram p19: hidden frame]
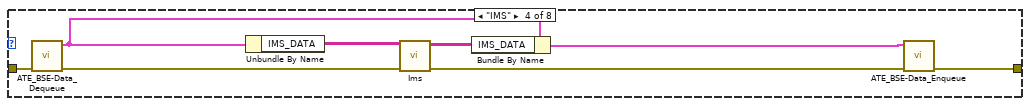
[diagram p20: hidden frame]
diagram:
  n1 = flat-sequence {
    tunnel: "Error In" -> [w6]
    tunnel: [w5] -> w1
    frame #0 {
      n2 = control-ref of="This VI"() -> (w4:refnum<vi>)
      n3 = invoke class="VI" method="Default Vals.Reinit All"(reference=w4, error in=w6) -> (reference out=w7:refnum<vi>, error out=w8:errorcluster)  [unwired: 1 in, 1 out]
      n4 = global write "ATE_GE_Manual Mode_VI Ref Global Variable.vi" "BSE"(w4) -> ()
      n5 = Close Reference(reference=w7, error in (no error)=w8) -> (error out=w5:errorcluster)
    }
  }
  n6 = case shown="No Error" w1 {
    selector: w1 -> [w18 w225]
    tunnel: [w23 w225] -> w3
    frame No Error {
      n7 = call "ATE_BSE_Event Queue FGV.vi"("Operations"=ATE_BSE_Queue_Operations."Init", "error in (no error)"=w18, "Queue name"="Event_Queue") -> ("error out"=w32:errorcluster)  [unwired: 7 in, 1 out]
      n8 = call "ATE_BSE_Data Queue FGV.vi"("Operations"=ATE_BSE_Queue_Operations."Init", "error in (no error)"=w32, "Queue name"="Data_Queue") -> ("error out"=w19:errorcluster)  [unwired: 7 in, 1 out]
      n9 = call "ATE_BSE-Data_Enqueue.vi"("error in (no error)"=w19, "element"=T21 {"Ref_Cluster"={"UE1"=refnum, "UE2"=refnum, "UE3"=refnum, "SelectNetwork1"=refnum, "SelectNetwork3"=refnum, "SelectNetwork2"=refnum, "Trace_Table1"=refnum, "UE - 1"=refnum, "UE - 2"=refnum, "UE - 3"=refnum, "UE - 4"=refnum, "Network-3"=refnum, "Status"=refnum, "Trace_Table2"=refnum, "UE4"=refnum, "Stop"=refnum, "Reset"=refnum, "IP simulation"=refnum, "Upload"=refnum, "Download"=refnum, "Network-1"=refnum, "Time Stamp"=refnum, "Network-2"=refnum, "IMS"=refnum, "GSM-Data"=refnum, "Configurations"=refnum, "Band"=refnum, "Sim Configurations"=refnum, "ECall"=refnum, "WWW"=refnum, "Cancel Configurations"=refnum, "GSM-PHY"=refnum, "GSM-CELL"=refnum, "GSM-GPRS"=refnum, "LTE-CELL"=refnum, "LTE-PHY"=refnum, "LTE-RRC"=refnum, "LTE-SDR"=refnum, "NR-RRC"=refnum, "NR-SDR"=refnum, "NR-PHY"=refnum, "NR-CELL"=refnum, "GSM-SDR"=refnum, "gNodeB-Data"=refnum, "eNodeB-Data"=refnum}, "Time Stamp"=timestamp(0 s since 1904-01-01), "Network-3"={"NW3-Thr-Down"=0.0, "NW3-Thr-Up"=0.0, "NW3-Fre-Down"=0.0, "NW3-Fre-Up"=0.0, "NW3-PwL-Down"=0.0, "NW3-PwL-Up"=0.0}, "Network-2"={"NW2-Thr-Down"=0.0, "NW2-Thr-Up"=0.0, "NW2-Fre-Down"=0.0, "NW2-Fre-Up"=0.0, "NW2-PwL-Down"=0.0, "NW2-PwL-Up"=0.0}, "Network-1"={"NW1-Thr-Down"=0.0, "NW1-Thr-Up"=0.0, "NW1-Fre-Down"=0.0, "NW1-Fre-Up"=0.0, "NW1-PwL-Down"=0.0, "NW1-PwL-Up"=0.0}, "UE - 4"={"UE4-Idle"=FALSE, "UE4-Origination"=FALSE, "UE4-Registration"=FALSE, "UE4-Pdu Connection"=FALSE, "UE4-Termination"=FALSE, "UE4-Detach"=FALSE}, "UE - 2"={"UE2-Idle"=FALSE, "UE2-Origination"=FALSE, "UE2-Registration"=FALSE, "UE2-Pdu Connection"=FALSE, "UE2-Termination"=FALSE, "UE2-Detach"=FALSE}, "UE - 1"={"UE1-Idle"=FALSE, "UE1-Origination"=FALSE, "UE1-Registration"=FALSE, "UE1-Pdu Connection"=FALSE, "UE1-Termination"=FALSE, "UE1-Detach"=FALSE}, "UE - 3"={"UE3-Idle"=FALSE, "UE3-Origination"=FALSE, "UE3-Registration"=FALSE, "UE3-Pdu Connection"=FALSE, "UE3-Termination"=FALSE, "UE3-Detach"=FALSE}, "IP simulation"=FALSE, "Stop"=FALSE, "Reset"=FALSE, "Download"=FALSE, "Upload"=FALSE, "UE4"=FALSE, "UE3"=FALSE, "UE2"=FALSE, "UE1"=FALSE, "Trace_Table1"=0, "Status"="", "Trace_Table2"=0, "SelectNetwork1"={"Nw1-check"=FALSE, "NW-Combo"="GSM"}, "SelectNetwork2"={"Nw1-check"=FALSE, "NW-Combo"="GSM"}, "SelectNetwork3"={"Nw1-check"=FALSE, "NW-Combo"="GSM"}, "IMS"=FALSE, "WWW"=FALSE, "Sim Configuration"=FALSE, "Ecall"=FALSE, "Configurations"=enum."Configurations", "Band"=enum."GSM", "GSM-Data"=enum."SDR", "eNodeB-Data"=enum."RRC", "gNodeB-Data"=enum."SDR", "Cancel Configurations"=FALSE, "GSM-SDR"={"DL Reference Power"=-13, "Serail Name"="", "UL Reference Power"=-13, "Radio Device"="0"}, "GSM-PHY"={"RACH Maximum Retransmission"="1", "RACH Transmission Slots"="14", "RACH Call Reestablishment"="1", "RACH Access Control Class"="0", "Block for Access Grant"="2", "Multiframe for Paging"="0", "Power Control Indicator"="0", "Radio Link Timeout"="15", "Cell Reselect Hysterisis"="3", "Attach/Detach Allowed"="1", "CCCH Combinations"="1", "t3212"=0, "DTX Indicator"="1", "Power Control Level"=0, "Minimum Received Signal Level"=0, "Half Rate Support"="0", "Add Reselect"="0"}, "GSM-CELL"={"SMS Enabled"="0", "Eutra Operating Bands"="850", "Power Offset Indicator"="0", "Early Classmark Sending Control"="0", "Location Area Code"=1, "CALL Enabled"="0", "Loop Back Enabled"="1", "GPRS Enabled"="0", "SI Type 2 ter Indicator"="1", "ARFCN"=0, "Frequency Format ID"=71, "Mobile Country Code"=1, "Mobile Network Code"=1, "Cell Barred Access"="0", "Downlink Frequency"=0, "Uplink Frequency"=900200000}, "GSM-GPRS"={"Priority Access THR"="6", "Acess Burst Type"="0", "Nack Countdown"="8", "BCCH/PDCH Measurement"="0", "Routing Area Code(RAC)"=128, "Network Control Order"="0", "t3168"="3", "t3192"="2", "Alpha"="10"}, "LTE-SDR"={"Radio Device"="0", "DL Reference Power"=-13, "Serail Name"="", "UL Reference Power"=-13, "DL Antennas"="1", "UL Antennas"="1"}, "LTE-PHY"={"PBCH Repetition"="0", "PUCCH Delta Shift"="1", "PUCCH CQI Number of RB"="0", "PHICH Resource"="ONESIXTH", "SRS Enable"="0", "PCCH Paging Cycle"="256", "BCCH Modification Coefficient"="2", "PUSCH Alpha"="1", "PUSCH DMRS Enable"="0", "PHICH Duration"="0", "PUCCH HARQ Max Transmission"=4, "PCCH Narrowband Count"="2", "PUSCH Power Offset"=-96, "PUCCH Power Offset"=-96, "PDSCH Power Boost"="0", "PUCCH An Occassions"="0", "PUUCH CS Antenna Ports"="1", "PRACH Response Window Size"="10", "PRACH Contention Resolution Timer"="48", "PRACH Ramping Step Size"="4", "PDSCH Reference Power"=-27, "PRACH Root Sequence Index"=0, "PRACH Maximum Transmissions"="10", "PRACH Initial Received Target Power"="-108", "PRACH Configuration Index"=0}, "LTE-CELL"={"Duplex Mode"="0", "Measurement Report"="1", "Eutra Operating Bands"="3", "Carrier Bandwidth"="10", "Physical Cell ID"=0, "Network Name"="MaxEye", "DL Frequency"=1842, "UL Frequency"=1747, "Transmission Mode"="TM1", "MNC Length"="2", "IMS Enabled"="0", "Tracking Area Code"=1, "Mobile Network Code"=1, "Mobile Country Code"=1}, "LTE-RRC"={"RLC Maximum Retransmision Threshold"="4", "RLC Timer Poll Retransmit"=80, "RLC Timer Reordering"=35, "RLC Timer Status Prohibit"=0, "RLC Poll PDU"=4, "RLC Poll Byte"=25}, "NR-SDR"={"DL Reference Power"=-13, "Serail Name"="", "UL Reference Power"=-13, "DL Antennas"="1", "UL Antennas"="1", "Radio Device"="0"}, "NR-PHY"={"PDSCH Reference Power"=-27, "SSB RSRP Threshold"=-109, "PRACH Contention Resolution Timer"=7, "Preamble Per SSB"=14, "Preamble Per SSB Format"=4, "UE Power Level Grant"=-90, "RA Response Window"="10", "Power Ramp Step Size"="2", "Preamble Root Sequence Index"="139", "Preamble Transmission Count"="10", "Preamble Received Power"=-96, "Zero Correlation Zone Configuration"=13, "Msg Frequency Division Multiplexing"="one", "PRACH Configuration Index"=98, "Preamble Timing Offset"=1, "Preamble Format"=0, "Resource Restriction Type"="0"}, "NR-CELL"={"Tracking Area Code"=1, "Mobile Country Code"=1, "Mobile Network Code"=1, "Operating Bands"="77", "Physical Cell ID"=0, "DL Offset to Carrier"=0, "Subcarrier Spacing"="1", "UL Offset to Carrier 2"=0, "Carrier Bandwidth"="10", "Transmission Mode"="TM1", "CSI-RS"="1", "SRS"="1", "Measurement Report"="1"}, "NR-RRC"={"Ciphering Algorithms for SRB"="0", "Integrity Algorithms for SRB"="0", "Ciphering Algorithms for DRB"="1", "Integrity Algorithms for DRB"="1"}, "IP_UI"={"Add"=FALSE, "Close"=FALSE, "IP_UI"=[]}, "IMS_DATA"=[], "ECall DATA"=[]} ("BSE_CONFIG")) -> ("error out"=w31:errorcluster)  [unwired: 9 in]
      n10 = call "ATE_BSE-Event_Enqueue.vi"("error in (no error)"=w31, "Event"=ATE_BSE_Event_type_def."Initialize") -> ("error out"=w17:errorcluster)  [unwired: 9 in]
      n11 = call "ATE_BSE-Data_Dequeue.vi"("error in (no error)"=w17) -> ("error out"=w16:errorcluster, "BSE_CONFIG"=w10:T21)  [unwired: 9 in]
      n12 = stacked-sequence {
        seq-local: [w35 _] -> [_ w70]
        tunnel: w10 -> [w36 _]
        tunnel: [_ w69] -> w9
        frame #0 {
          n13 = control-ref of="Trace_Table1"() -> (w51:refnum<vi>)
          n14 = control-ref of="Trace_Table2"() -> (w50:refnum<vi>)
          n15 = control-ref of="eNodeB-Data"() -> (w34:refnum<vi>)
          n16 = control-ref of="gNodeB-Data"() -> (w33:refnum<vi>)
          n17 = control-ref of="GSM-Data"() -> (w43:refnum<vi>)
          n18 = control-ref of="Configurations"() -> (w41:refnum<vi>)
          n19 = control-ref of="Band"() -> (w42:refnum<vi>)
          n20 = control-ref of="Time Stamp"() -> (w64:refnum<vi>)
          n21 = control-ref of="Download"() -> (w59:refnum<vi>)
          n22 = control-ref of="IP simulation"() -> (w58:refnum<vi>)
          n23 = control-ref of="Reset"() -> (w57:refnum<vi>)
          n24 = control-ref of="Start"() -> (w56:refnum<vi>)
          n25 = control-ref of="Upload"() -> (w55:refnum<vi>)
          n26 = control-ref of="UE1"() -> (w54:refnum<vi>)
          n27 = control-ref of="UE2"() -> (w53:refnum<vi>)
          n28 = control-ref of="UE3"() -> (w45:refnum<vi>)
          n29 = control-ref of="UE4"() -> (w52:refnum<vi>)
          n30 = control-ref of="Sim Configurations"() -> (w40:refnum<vi>)
          n31 = control-ref of="ECall"() -> (w39:refnum<vi>)
          n32 = control-ref of="WWW"() -> (w38:refnum<vi>)
          n33 = control-ref of="IMS"() -> (w44:refnum<vi>)
          n34 = control-ref of="Cancel Configurations"() -> (w37:refnum<vi>)
          n35 = control-ref of="Network-1"() -> (w67:refnum<vi>)
          n36 = control-ref of="Network-2"() -> (w66:refnum<vi>)
          n37 = control-ref of="Network-3"() -> (w65:refnum<vi>)
          n38 = control-ref of="UE - 1"() -> (w63:refnum<vi>)
          n39 = control-ref of="UE - 2"() -> (w62:refnum<vi>)
          n40 = control-ref of="UE - 3"() -> (w61:refnum<vi>)
          n41 = control-ref of="UE - 4"() -> (w60:refnum<vi>)
          n42 = control-ref of="SelectNetwork1"() -> (w48:refnum<vi>)
          n43 = control-ref of="SelectNetwork2"() -> (w47:refnum<vi>)
          n44 = control-ref of="SelectNetwork3"() -> (w46:refnum<vi>)
          n45 = control-ref of="Status"() -> (w49:refnum<vi>)
          n46 = Bundle By Name(cluster=w36, "Ref_Cluster.Network-1"=w67, "Ref_Cluster.Network-2"=w66, "Ref_Cluster.Network-3"=w65, "Ref_Cluster.Time Stamp"=w64, "Ref_Cluster.UE - 1"=w63, "Ref_Cluster.UE - 2"=w62, "Ref_Cluster.UE - 3"=w61, "Ref_Cluster.UE - 4"=w60, "Ref_Cluster.Download"=w59, "Ref_Cluster.IP simulation"=w58, "Ref_Cluster.Reset"=w57, "Ref_Cluster.Stop"=w56, "Ref_Cluster.Upload"=w55, "Ref_Cluster.UE1"=w54, "Ref_Cluster.UE2"=w53, "Ref_Cluster.UE3"=w45, "Ref_Cluster.UE4"=w52, "Ref_Cluster.Trace_Table1"=w51, "Ref_Cluster.Trace_Table2"=w50, "Ref_Cluster.Status"=w49, "Ref_Cluster.SelectNetwork1"=w48, "Ref_Cluster.SelectNetwork2"=w47, "Ref_Cluster.SelectNetwork3"=w46, "Ref_Cluster.Sim Configurations"=w40, "Ref_Cluster.ECall"=w39, "Ref_Cluster.WWW"=w38, "Ref_Cluster.IMS"=w44, "Ref_Cluster.GSM-Data"=w43, "Ref_Cluster.eNodeB-Data"=w34, "Ref_Cluster.gNodeB-Data"=w33, "Ref_Cluster.Configurations"=w41, "Ref_Cluster.Band"=w42, "Ref_Cluster.Cancel Configurations"=w37) -> (w35:T21)
        }
        frame #1 {
          n47 = control-ref of="GSM-SDR"() -> (w68:refnum<vi>)
          n48 = control-ref of="GSM-GPRS"() -> (w81:refnum<vi>)
          n49 = control-ref of="GSM-CELL"() -> (w80:refnum<vi>)
          n50 = control-ref of="GSM-PHY"() -> (w79:refnum<vi>)
          n51 = control-ref of="LTE-SDR"() -> (w78:refnum<vi>)
          n52 = control-ref of="LTE-PHY"() -> (w77:refnum<vi>)
          n53 = control-ref of="LTE-CELL"() -> (w76:refnum<vi>)
          n54 = control-ref of="LTE-RRC"() -> (w75:refnum<vi>)
          n55 = control-ref of="NR-SDR"() -> (w74:refnum<vi>)
          n56 = control-ref of="NR-CELL"() -> (w73:refnum<vi>)
          n57 = control-ref of="NR-PHY"() -> (w72:refnum<vi>)
          n58 = control-ref of="NR-RRC"() -> (w71:refnum<vi>)
          n59 = Bundle By Name(cluster=w70, "Ref_Cluster.GSM-SDR"=w68, "Ref_Cluster.GSM-GPRS"=w81, "Ref_Cluster.GSM-CELL"=w80, "Ref_Cluster.GSM-PHY"=w79, "Ref_Cluster.LTE-SDR"=w78, "Ref_Cluster.LTE-PHY"=w77, "Ref_Cluster.LTE-CELL"=w76, "Ref_Cluster.LTE-RRC"=w75, "Ref_Cluster.NR-SDR"=w74, "Ref_Cluster.NR-CELL"=w73, "Ref_Cluster.NR-PHY"=w72, "Ref_Cluster.NR-RRC"=w71) -> (w69:T21)
        }
      }
      n60 = call "ATE_BSE-Data_Enqueue.vi"("error in (no error)"=w16, "element"=w9) -> ("error out"=w15:errorcluster)  [unwired: 9 in]
      n61 = disable-structure shown="Disabled" {
        frame Disabled {
          n62 = call "ATE_BSE-Data_Dequeue.vi"() -> ()  [unwired: 10 in, 2 out]
          n63 = call "ATE_BSE-Event_Dequeue.vi"() -> ()  [unwired: 10 in, 2 out]
          n64 = call "ATE_BSE-Data_Enqueue.vi"() -> ()  [unwired: 11 in, 1 out]
          n65 = call "ATE_BSE-Event_Enqueue.vi"() -> ()  [unwired: 11 in, 1 out]
        }
        frame Enabled {
        }
      }
      n66 = call "Exit_Event_Handlervi.vi"("error in (no error)"=w15, "Exit?"=FALSE, "Command"=Exit_Event_Handle_Comamnd."Init" ("Enum")) -> ("error out"=w26:errorcluster, "Event Registration Refnum out"=w30:refnum<event-registration>)  [unwired: 6 in, 1 out]
      n67 = while {
        tunnel: w30 -> [w83]
        tunnel: [w82] -> w28
        tunnel: w26 -> [w86]
        tunnel: [w85] -> w29
        stop <- w87 stop-if-true
        # "Producer Loop - Capture the Event"
        n68 = event shown="[10] \"Start\": Value Change" {
          selector: w83 -> [_ _ _ _ _ _ _ _ _ _ _ _ _]
          dyn-events: [_ _ _ _ _ _ _ _ _ _ _ _ _] -> w82
          timeout: 10 -> [_ _ _ _ _ _ _ _ _ _ _ _ _]
          tunnel: [_ _ _ _ _ _ _ _ _ _ _ TRUE w166] -> w87
          tunnel: w86 -> [w88 w100 w119 w128 w137 w138 w142 w145 w148 w151 w154 w157 w163]
          tunnel: [w88 w99 w118 w127 w136 w139 w143 w146 w149 w150 w153 w158 w164] -> w85
          event Timeout {
            n69 = event-data() -> ()  [unwired: 1 in, 1 out]
          }
          event "SelectNetwork1", "SelectNetwork2", "SelectNetwork3": Mouse Down {
            n70 = event-data() -> ("Time"=w96:u32, "CtlRef"=w93:refnum<vi>)  [unwired: 1 in]
            n71 = call "ATE_BSE-Data_Dequeue.vi"("error in (no error)"=w100) -> ("error out"=w98:errorcluster, "BSE_CONFIG"=w94:T21)  [unwired: 9 in]
            n72 = call "Double Click.vi"("Time"=w96) -> ("Double Click"=w91:bool)  [unwired: 10 in]
            n73 = call "Select Network.vi"("BSE_CONFIG"=w94, "Current Reference"=w93) -> ("NW-Combo"=w89:string, "Nw-check"=w90:bool)  [unwired: 8 in]
            n74 = And(x=w91, y=w90) -> (x .and. y?=w92:bool)
            n75 = case shown="False" w92 {
              tunnel: w98 -> [w102 w109]
              tunnel: [w102 w103] -> w97
              tunnel: w94 -> [w101 w110]
              tunnel: [w101 w110] -> w95
              tunnel: w89 -> [_ w106]
              frame False {
              }
              frame True {
                n76 = Search 1D Array(1D array=string[] ["GSM", "eNodeB", "gNodeB"], element=w106) -> (index of element=w105:i32)  [unwired: 1 in]
                n77 = property on="Configurations" class="TabCtl (strict)"(error in=w109, "Value"=enum32{"Configurations", "Main"}."Configurations" ("Configurations")) -> (error out=w104:errorcluster)  [unwired: 1 in, 1 out]
                n78 = property on="Band" class="TabCtl (strict)"(error in=w104, "Value"=w105) -> (error out=w103:errorcluster)  [unwired: 1 in, 1 out]
              }
            }
            n79 = call "ATE_BSE-Data_Enqueue.vi"("error in (no error)"=w97, "element"=w95) -> ("error out"=w99:errorcluster)  [unwired: 9 in]
          }
          event "GSM-SDR", "GSM-CELL", "GSM-GPRS", "GSM-PHY": Value Change {
            n80 = event-data() -> ()  [unwired: 1 in, 6 out]
            n81 = call "ATE_BSE-Data_Dequeue.vi"("error in (no error)"=w119) -> ("error out"=w115:errorcluster, "BSE_CONFIG"=w116:T21)  [unwired: 9 in]
            n82 = Bundle By Name(cluster=w116, "GSM-SDR"="GSM-SDR", "GSM-PHY"="GSM-PHY", "GSM-CELL"="GSM-CELL", "GSM-GPRS"="GSM-GPRS") -> (w117:T21)
            n83 = call "ATE_BSE-Data_Enqueue.vi"("error in (no error)"=w115, "element"=w117) -> ("error out"=w118:errorcluster)  [unwired: 9 in]
          }
          event "LTE-SDR", "LTE-CELL", "LTE-PHY", "LTE-RRC": Value Change {
            n84 = event-data() -> ()  [unwired: 1 in, 6 out]
            n85 = call "ATE_BSE-Data_Dequeue.vi"("error in (no error)"=w128) -> ("error out"=w124:errorcluster, "BSE_CONFIG"=w125:T21)  [unwired: 9 in]
            n86 = Bundle By Name(cluster=w125, "LTE-SDR"="LTE-SDR", "LTE-PHY"="LTE-PHY", "LTE-CELL"="LTE-CELL", "LTE-RRC"="LTE-RRC") -> (w126:T21)
            n87 = call "ATE_BSE-Data_Enqueue.vi"("error in (no error)"=w124, "element"=w126) -> ("error out"=w127:errorcluster)  [unwired: 9 in]
          }
          event "NR-SDR", "NR-CELL", "NR-PHY", "NR-RRC": Value Change {
            n88 = event-data() -> ()  [unwired: 1 in, 6 out]
            n89 = call "ATE_BSE-Data_Dequeue.vi"("error in (no error)"=w137) -> ("error out"=w133:errorcluster, "BSE_CONFIG"=w134:T21)  [unwired: 9 in]
            n90 = Bundle By Name(cluster=w134, "NR-SDR"="NR-SDR", "NR-PHY"="NR-PHY", "NR-CELL"="NR-CELL", "NR-RRC"="NR-RRC") -> (w135:T21)
            n91 = call "ATE_BSE-Data_Enqueue.vi"("error in (no error)"=w133, "element"=w135) -> ("error out"=w136:errorcluster)  [unwired: 9 in]
          }
          event "Cancel Configurations": Value Change {
            n92 = event-data() -> ()  [unwired: 1 in, 6 out]
            n93 = property on="Configurations" class="TabCtl (strict)"(error in=w138, "Value"=enum32{"Configurations", "Main"}."Main" ("Configurations")) -> (error out=w139:errorcluster)  [unwired: 1 in, 1 out]
          }
          event "Configure": Value Change {
            n94 = event-data() -> ()  [unwired: 1 in, 6 out]
            n95 = call "ATE_BSE-Event_Enqueue.vi"("error in (no error)"=w142, "Event"=ATE_BSE_Event_type_def."Configure") -> ("error out"=w143:errorcluster)  [unwired: 9 in]
          }
          event "IMS": Value Change {
            n96 = event-data() -> ()  [unwired: 1 in, 6 out]
            n97 = call "ATE_BSE-Event_Enqueue.vi"("error in (no error)"=w145, "Event"=ATE_BSE_Event_type_def."IMS") -> ("error out"=w146:errorcluster)  [unwired: 9 in]
          }
          event "ECall": Value Change {
            n98 = event-data() -> ()  [unwired: 1 in, 6 out]
            n99 = call "ATE_BSE-Event_Enqueue.vi"("error in (no error)"=w148, "Event"=ATE_BSE_Event_type_def."ECall") -> ("error out"=w149:errorcluster)  [unwired: 9 in]
          }
          event "IP simulation": Value Change {
            n100 = event-data() -> ()  [unwired: 1 in, 6 out]
            n101 = call "ATE_BSE-Event_Enqueue.vi"("error in (no error)"=w151, "Event"=ATE_BSE_Event_type_def."Ip Simulation") -> ("error out"=w150:errorcluster)  [unwired: 9 in]
          }
          event "Start": Value Change {
            n102 = event-data() -> ()  [unwired: 1 in, 6 out]
            n103 = call "ATE_BSE-Event_Enqueue.vi"("error in (no error)"=w154, "Event"=ATE_BSE_Event_type_def."Ip Simulation") -> ("error out"=w153:errorcluster)  [unwired: 9 in]
          }
          event User Event {
            n104 = event-data() -> ()  [unwired: 1 in, 5 out]
            n105 = call "ATE_BSE_Event Queue FGV.vi"("Operations"=ATE_BSE_Queue_Operations."Close", "error in (no error)"=w157) -> ("error out"=w158:errorcluster)  [unwired: 8 in, 1 out]
          }
          event Panel Close? {
            w166 = TRUE
            n106 = event-data() -> ()  [unwired: 1 in, 4 out]
            n107 = call "ATE_BSE-Data_Dequeue.vi"("error in (no error)"=w163) -> ("error out"=w162:errorcluster, "BSE_CONFIG"=w160:T21)  [unwired: 9 in]
            n108 = call "ATE_BSE-Data_Enqueue.vi"("error in (no error)"=w162, "element"=w160) -> ("error out"=w161:errorcluster)  [unwired: 9 in]
            n109 = call "ATE_BSE_Event Queue FGV.vi"("Operations"=ATE_BSE_Queue_Operations."Close", "error in (no error)"=w161) -> ("error out"=w164:errorcluster)  [unwired: 8 in, 1 out]
            n110 = event-data("Discard?"=w166) -> ()  [unwired: 1 in, 1 out]
          }
        }
      }
      n111 = while {
        tunnel: w26 -> [w168]
        tunnel: [w171] -> w24
        stop <- w170 stop-if-true
        # "Consumer Loop - Processes the Events"
        n112 = call "ATE_BSE-Event_Dequeue.vi"("error in (no error)"=w168) -> ("error out"=w169:errorcluster, "Event"=w167:T26)  [unwired: 9 in]
        n113 = case shown="\"Start Base Station\"" w167 {
          tunnel: w169 -> [w178 w189 w197 w205 w213 w221 w222 w224]
          tunnel: [w180 w188 w196 w204 w212 w220 w222 w224] -> w171
          tunnel: [_ _ _ _ _ _ TRUE _] -> w170
          frame "Initialize" {
            n114 = call "ATE_BSE-Data_Dequeue.vi"("error in (no error)"=w178) -> ("error out"=w172:errorcluster, "BSE_CONFIG"=w175:T21)  [unwired: 9 in]
            n115 = Bundle By Name(cluster=w175, "IP_UI.IP_UI"=T28 []) -> (w174:T21)
            n116 = call "TCP_FGV.vi"("error in (no error)"=w172, "Operation"=TCP_FGV."Open") -> ("error out"=w177:errorcluster)  [unwired: 7 in, 1 out]
            n117 = call <vilib>:"Clear Errors.vi"("error in (no error)"=w177) -> ("error out"=w176:errorcluster)  [unwired: 5 in, 1 out]
            n118 = call "ATE_BSE-Data_Enqueue.vi"("error in (no error)"=w176, "element"=w174) -> ("error out"=w180:errorcluster)  [unwired: 9 in]
          }
          frame "Configure" {
            n119 = call "ATE_BSE-Data_Dequeue.vi"("error in (no error)"=w189) -> ("error out"=w187:errorcluster, "BSE_CONFIG"=w184:T21)  [unwired: 9 in]
            n120 = property on="Band" class="TabCtl (strict)"(error in=w187) -> (error out=w186:errorcluster, "Value"=w183:enum32{"GSM", "eNodeB", "gNodeB"})  [unwired: 1 in, 1 out]
            n121 = call "Configure_Run.vi"("error in"=w186, "Base Station"=T30 "BS1", "Band"=w183, "Input"=w184) -> ("error out"=w185:errorcluster)  [unwired: 7 in]
            n122 = call <vilib>:"Clear Errors.vi"("error in (no error)"=w185) -> ("error out"=w182:errorcluster)  [unwired: 5 in, 1 out]
            n123 = call "ATE_BSE-Data_Enqueue.vi"("error in (no error)"=w182, "element"=w184) -> ("error out"=w188:errorcluster)  [unwired: 9 in]
          }
          frame "Ip Simulation" {
            n124 = call "ATE_BSE-Data_Dequeue.vi"("error in (no error)"=w197) -> ("error out"=w193:errorcluster, "BSE_CONFIG"=w191:T21)  [unwired: 9 in]
            n125 = Unbundle By Name(w191) -> ("IP_UI"=w195:T31)
            n126 = call "IP_Simulation.vi"("error constant"=w193, "IP_UI"=w195) -> ("error constant"=w192:errorcluster, "Out"=w194:T31)  [unwired: 8 in]
            n127 = Bundle By Name(cluster=w191, "IP_UI"=w194) -> (w190:T21)
            n128 = call "ATE_BSE-Data_Enqueue.vi"("error in (no error)"=w192, "element"=w190) -> ("error out"=w196:errorcluster)  [unwired: 9 in]
          }
          frame "IMS" {
            n129 = call "ATE_BSE-Data_Dequeue.vi"("error in (no error)"=w205) -> ("error out"=w203:errorcluster, "BSE_CONFIG"=w200:T21)  [unwired: 9 in]
            n130 = Unbundle By Name(w200) -> ("IMS_DATA"=w201:string[][])
            n131 = call "Ims.vi"("error in (no error)"=w203, "IMS 2"=w201) -> ("error out"=w202:errorcluster, "IMS"=w199:string[][])  [unwired: 6 in]
            n132 = Bundle By Name(cluster=w200, "IMS_DATA"=w199) -> (w198:T21)
            n133 = call "ATE_BSE-Data_Enqueue.vi"("error in (no error)"=w202, "element"=w198) -> ("error out"=w204:errorcluster)  [unwired: 9 in]
          }
          frame "ECall" {
            n134 = call "ATE_BSE-Data_Dequeue.vi"("error in (no error)"=w213) -> ("error out"=w211:errorcluster, "BSE_CONFIG"=w207:T21)  [unwired: 9 in]
            n135 = Unbundle By Name(w207) -> ("ECall DATA"=w209:string[][])
            n136 = call "ECall.vi"("error in (no error)"=w211, "ECall"=w209) -> ("error out"=w210:errorcluster, "ECall"=w208:string[][])  [unwired: 6 in]
            n137 = Bundle By Name(cluster=w207, "ECall DATA"=w208) -> (w206:T21)
            n138 = call "ATE_BSE-Data_Enqueue.vi"("error in (no error)"=w210, "element"=w206) -> ("error out"=w212:errorcluster)  [unwired: 9 in]
          }
          frame "Start Base Station" {
            n139 = call "ATE_BSE-Data_Dequeue.vi"("error in (no error)"=w221) -> ("error out"=w219:errorcluster, "BSE_CONFIG"=w215:T21)  [unwired: 9 in]
            n140 = Unbundle By Name(w215) -> ("ECall DATA"=w217:string[][])
            n141 = call "ECall.vi"("error in (no error)"=w219, "ECall"=w217) -> ("error out"=w218:errorcluster, "ECall"=w216:string[][])  [unwired: 6 in]
            n142 = Bundle By Name(cluster=w215, "ECall DATA"=w216) -> (w214:T21)
            n143 = call "ATE_BSE-Data_Enqueue.vi"("error in (no error)"=w218, "element"=w214) -> ("error out"=w220:errorcluster)  [unwired: 9 in]
          }
          frame "Exit" {
          }
          frame "Error" {
          }
        }
      }
      n144 = Unregister For Events(event registration refnum=w28, error in=w29) -> (error out=w25:errorcluster)
      n145 = Merge Errors(w25, w24) -> (w23:errorcluster)
    }
    frame Error {
    }
  }
  "Error Out" <- w3
